vi "GetYAxisList.vi"(8 "error in (no error)":errorcluster caption="エラー入力（エラーなし）", 10 "ChName[]":string[](array[string]), 11 "波形グラフref":refnum<vi>) -> (0 "error out":errorcluster caption="エラー出力", 2 "X軸名称[]":string[](array[string]), 3 "Y軸名称[]":string[](array[string]), 4 "グラフ表示?[]":bool[](array[boolean]), 5 "Y軸ref[]":refnum<vi>[](array[refnum]), 7 "X軸ref[]":refnum<vi>[](array[refnum]))   [LabVIEW 2014]
uses:
  GlobalData/GlobalData.vi
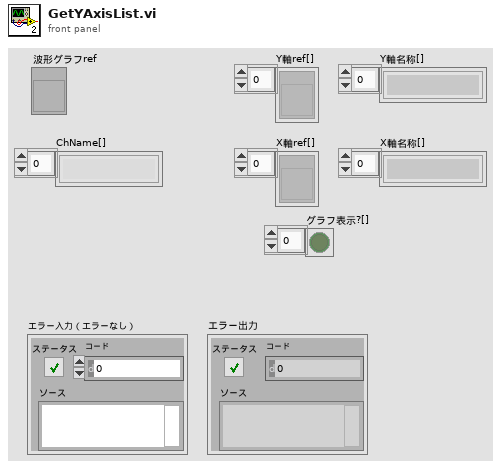
[diagram p1: front panel]
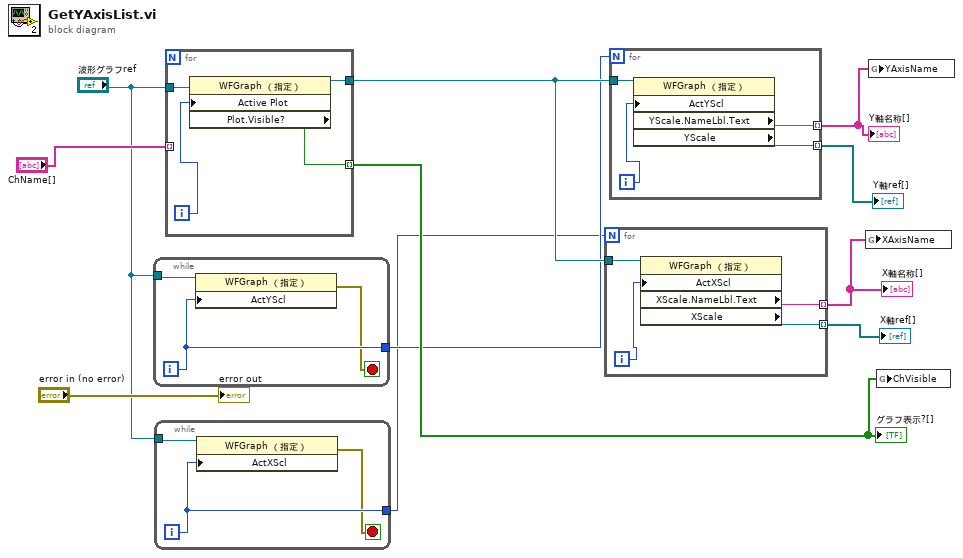
[diagram p0: block diagram]
diagram:
  n1 = while {
    tunnel: "波形グラフref" -> [w14]
    tunnel: [w13] -> w3
    i -> [w13]
    stop <- w12 stop-if-true
    n2 = property class="WFGraph （指定）"(reference=w14, "ActYScl"=w13) -> (error out=w12:errorcluster)  [unwired: 1 in, 1 out]
  }
  n3 = while {
    tunnel: "波形グラフref" -> [w17]
    tunnel: [w16] -> w1
    i -> [w16]
    stop <- w15 stop-if-true
    n4 = property class="WFGraph （指定）"(reference=w17, "ActXScl"=w16) -> (error out=w15:errorcluster)  [unwired: 1 in, 1 out]
  }
  n5 = for {
    tunnel: "ChName[]" -> [_] mode=indexing
    tunnel: "波形グラフref" -> [w21]
    tunnel: [w19] -> w9
    tunnel: [w18] -> w4 mode=indexing
    i -> [w20]
    n6 = property class="WFGraph （指定）"(reference=w21, "Active Plot"=w20) -> (reference out=w19:refnum<vi>, "Plot.Visible?"=w18:bool)  [unwired: 1 in, 1 out]
  }
  "グラフ表示?[]" <- w4
  n7 = for {
    N: w1 -> [_]
    tunnel: w9 -> [w25]
    tunnel: [w24] -> w6 mode=indexing
    tunnel: [w23] -> w7 mode=indexing
    i -> [w22]
    n8 = property class="WFGraph （指定）"(reference=w25, "ActXScl"=w22) -> ("XScale.NameLbl.Text"=w24:string, "XScale"=w23:refnum<vi>)  [unwired: 1 in, 2 out]
  }
  "X軸ref[]" <- w7
  "X軸名称[]" <- w6
  n9 = for {
    N: w3 -> [_]
    tunnel: w9 -> [w29]
    tunnel: [w28] -> w10 mode=indexing
    tunnel: [w27] -> w11 mode=indexing
    i -> [w26]
    n10 = property class="WFGraph （指定）"(reference=w29, "ActYScl"=w26) -> ("YScale.NameLbl.Text"=w28:string, "YScale"=w27:refnum<vi>)  [unwired: 1 in, 2 out]
  }
  "Y軸名称[]" <- w10
  "Y軸ref[]" <- w11
  n11 = global write "GlobalData.vi" "XAxisName"(w6) -> ()
  n12 = global write "GlobalData.vi" "YAxisName"(w10) -> ()
  n13 = global write "GlobalData.vi" "ChVisible"(w4) -> ()
  "error out" <- "error in (no error)"
